vi "Example_Save or Load Controls To From File.vi"() -> ()   [LabVIEW 2020]
doc: "Demonstrates how GUI object values can be saved into configuration file or loaded from the configuration file. This feature is extremely useful to manage settings of the application. Another, and very important, feature is that adding or removing items to be saved is taking minimum time."
uses:
  VI Server Toolkit LV2013.lvlib
  <vilib>/Utility/config.llb/NI_LVConfig.lvlib
  <vilib>/Utility/config.llb/Read Key (String).vi
panel:
  in  "2D Array - Boolean":bool[][](array[boolean]) caption="2D Array - String"
  in  "2D Array - Path":path[][](array[path]) caption="2D Array - String"
  in  "EXIT":bool
  out "LED":bool
  in  "Error In":errorcluster
  out "error out":errorcluster
  in  "SystemConfigurationFile":path=path "I:/Working Directory/Projects/VI Server Toolkit 2013 Distribution/VI Server ToolKit/VI Server_Examples/System Configuration.cfg" caption="System Configuration File"
  in  "Load":bool
  in  "Save":bool
  in  "2D Array - String":string[][](array[string])
  in  "2D Array - DBL":dbl[][](array[numeric])
  in  "Menu Ring":u16(ring) items=["Item 1", "Item 2", "Item 3"]
  in  "1D Array - DBL":dbl[](array[numeric])
  in  "1D Array - String":string[](array[string])
  in  "Settings Button":bool
  in  "Knob":dbl(knob) scale=0.0..10.0
  in  "Horizontal Fill Slide":dbl(slide) scale=0.0..10.0
  in  "Numeric Control":dbl
  # "INSTRUCTIONS:\n\n1. Create the \"System configuration\" file path.\n2. Populate array elements, set controls and ring selection.\n3. Save the settings into configuration file (SAVE button).\n4. Change settings, empty arrays.\n5. Press LOAD button and verify the settings are properly updated.\n6. Examine the block diagram and note the Control Labels array which contains \nall labels of the saved/loaded controls."
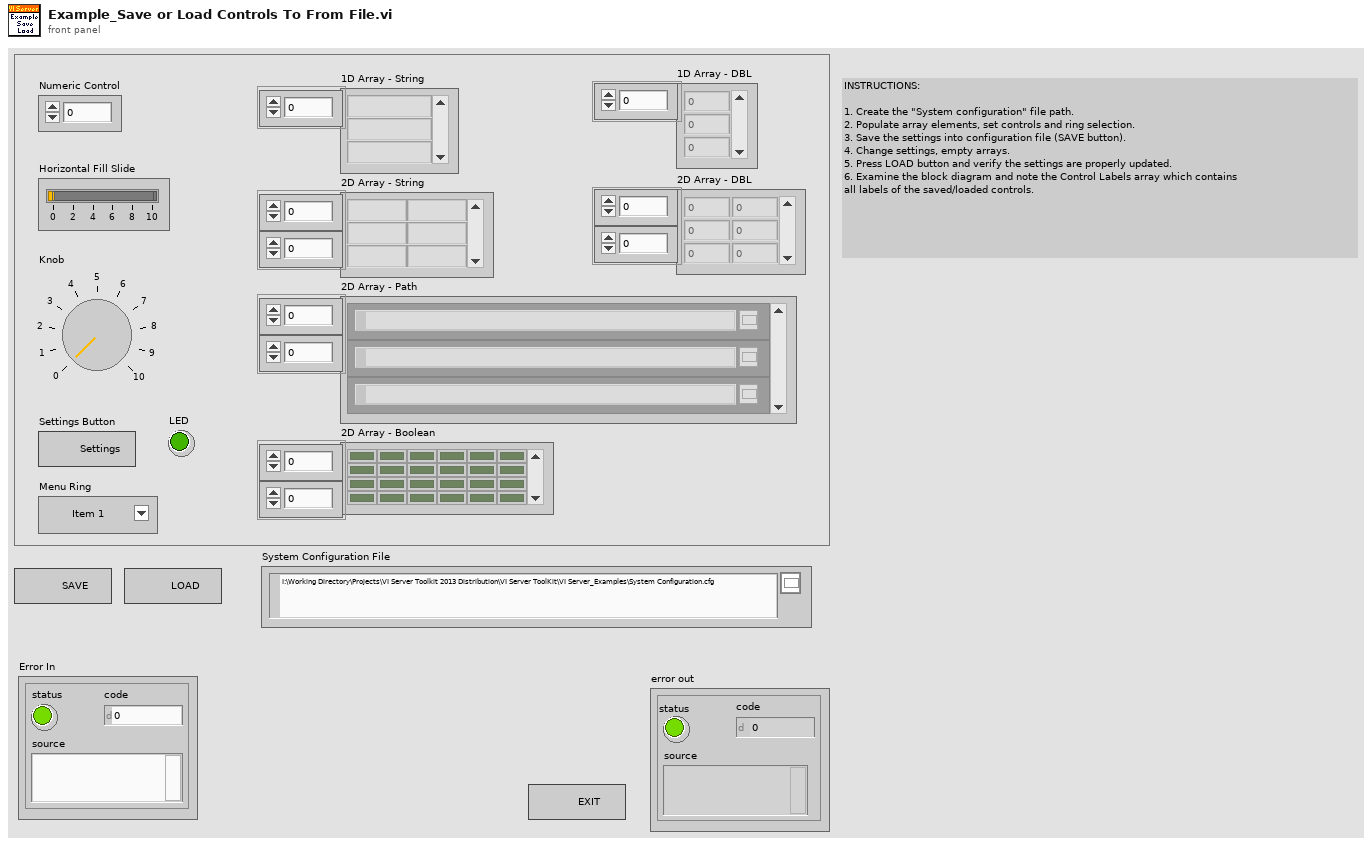
[diagram p1: front panel]
types:
  T1 = typedef "VI Server_RefsCluster.ctl" = cluster{"Labels":string[], "Refs":refnum<vi>[], "VI Ref":refnum<vi>}
  T2 = typedef "NI_LVConfig.lvlib/Config Data RefNum.ctl" = refnum<k1>
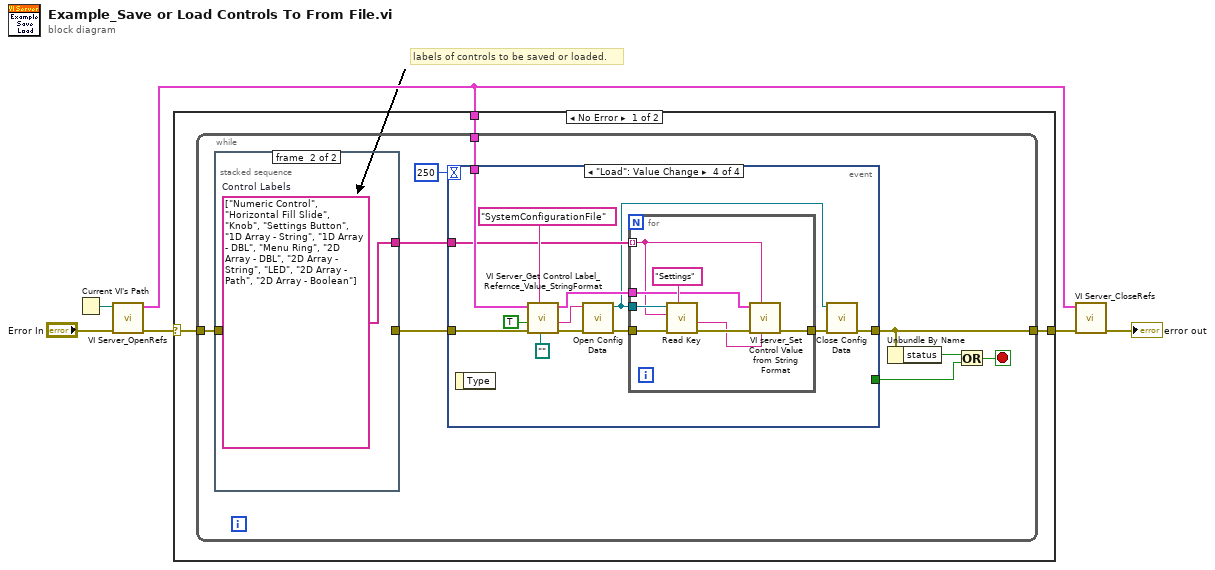
[diagram p0: block diagram]
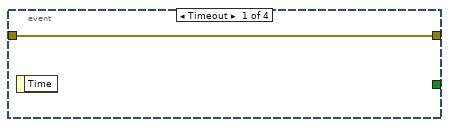
[diagram p2: hidden frame]
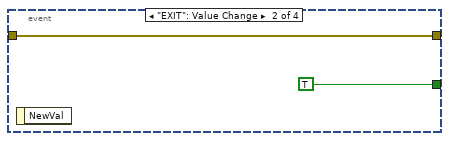
[diagram p3: hidden frame]
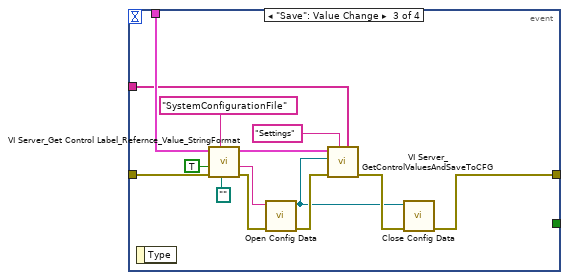
[diagram p4: hidden frame]
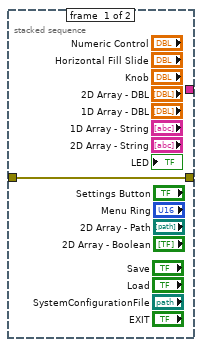
[diagram p5: hidden frame]
diagram:
  # "labels of controls to be saved or loaded."
  n1 = Current VI's Path() -> (path=w5:path)
  n2 = call "VI Server_OpenRefs.vi"("error in"="Error In", "VI Path"=w5) -> ("error out"=w4:errorcluster, "VI Server.RefsCluster"=w1:T1)  [unwired: 8 in]
  n3 = case shown="No Error" w4 {
    selector: w4 -> [w9 w59]
    tunnel: [w8 w59] -> w3
    tunnel: w1 -> [w7 _]
    frame No Error {
      n4 = while {
        tunnel: w9 -> [w17]
        tunnel: [w15] -> w8
        tunnel: w7 -> [w11]
        stop <- w12 stop-if-true
        n5 = stacked-sequence {
          tunnel: [w57 _] -> w16
          tunnel: w17 -> [w57 _]
          tunnel: [_ w58] -> w10
          frame #0 {
          }
          frame #1 {
            w58 = string[] ["Numeric Control", "Horizontal Fill Slide", "Knob", "Settings Button", "1D Array - String", "1D Array - DBL", "Menu Ring", "2D Array - DBL", "2D Array - String", "LED", "2D Array - Path", "2D Array - Boolean"]  # Control Labels
          }
        }
        n6 = event shown="[3] \"Load\": Value Change" {
          selector: _ -> [_ _ _ _]
          dyn-events: _ -> [_ _ _ _]
          timeout: 250 -> [_ _ _ _]
          tunnel: w16 -> [w19 w21 w28 w43]
          tunnel: [w19 w21 w23 w41] -> w15
          tunnel: [_ TRUE _ _] -> w13
          tunnel: w11 -> [_ _ w27 w42]
          tunnel: w10 -> [_ _ w26 w38]
          event Timeout {
            n7 = event-data() -> ()  [unwired: 1 in, 1 out]
          }
          event "EXIT": Value Change {
            n8 = event-data() -> ()  [unwired: 1 in, 1 out]
          }
          event "Save": Value Change {
            n9 = event-data() -> ()  [unwired: 1 in, 1 out]
            n10 = call "VI Server_Get Control Label_Refernce_Value_StringFormat.vi"(6:path "", "Label"="SystemConfigurationFile", "error in (no error)"=w28, 9:TRUE ("Single Instance (T)"), "VI Server Cluster"=w27) -> ("error out"=w31:errorcluster, "ControlValue(StringFormat)"=w32:string, "VI Server Cluster.DUP"=w29:T1)  [unwired: 4 in]
            n11 = call <vilib>:"Open Config Data.vi"("error in (no error)"=w31, "configuration file path"=w32) -> ("error out"=w30:errorcluster, "refnum"=w22:T2)  [unwired: 7 in, 1 out]
            n12 = call "VI Server_GetControlValuesAndSaveToCFG.vi"("Labels"=w26, "Section"="Settings", "error in"=w30, "CFG File.Ref"=w22, "VI Server Cluster"=w29) -> ("error out"=w24:errorcluster)  [unwired: 3 in, 3 out]
            n13 = call <vilib>:"Close Config Data.vi"("error in (no error)"=w24, "refnum"=w22) -> ("error out"=w23:errorcluster)  [unwired: 8 in, 1 out]
          }
          event "Load": Value Change {
            n14 = event-data() -> ()  [unwired: 1 in, 1 out]
            n15 = call "VI Server_Get Control Label_Refernce_Value_StringFormat.vi"(6:path "", "Label"="SystemConfigurationFile", "error in (no error)"=w43, 9:TRUE ("Single Instance (T)"), "VI Server Cluster"=w42) -> ("error out"=w44:errorcluster, "ControlValue(StringFormat)"=w45:string, "VI Server Cluster.DUP"=w37:T1)  [unwired: 4 in]
            n16 = call <vilib>:"Open Config Data.vi"("error in (no error)"=w44, "configuration file path"=w45) -> ("error out"=w40:errorcluster, "refnum"=w36:T2)  [unwired: 7 in, 1 out]
            n17 = for {
              tunnel: w40 -> [w56]
              tunnel: w36 -> [w54]
              tunnel: [w52] -> w39
              tunnel: w38 -> [w49] mode=indexing
              tunnel: w37 -> [w50]
              n18 = call-poly <vilib>:"Read Key.vi"("section"="Settings" ("Section"), "error in (no error)"=w56, "key"=w49, "refnum"=w54) -> ("error out"=w53:errorcluster, "value"=w51:string)  [unwired: 4 in, 2 out]
              n19 = call "VI server_Set Control Value from String Format.vi"("Value.STR"=w51, "Label"=w49, "error in (no error)"=w53, "VI Server Cluster"=w50) -> ("error out"=w52:errorcluster)  [unwired: 5 in, 2 out]
            }
            n20 = call <vilib>:"Close Config Data.vi"("error in (no error)"=w39, "refnum"=w36) -> ("error out"=w41:errorcluster)  [unwired: 8 in, 1 out]
          }
        }
        n21 = Unbundle By Name(w15) -> ("status"=w14:bool)
        n22 = Or(x=w14, y=w13) -> (x .or. y?=w12:bool)
      }
    }
    frame Error {
    }
  }
  n23 = call "VI Server_CloseRefs.vi"("error in"=w3, "VI Server.RefsCluster"=w1) -> ("error out"=→"error out":errorcluster)  [unwired: 9 in]
